vi "AddVIsToClass.vi"(8 "error in (no error)":errorcluster, 10 "Destination Folder":refnum<vi>, 11 "BaseAccessorScripter in":refnum<class "BaseAccessorScripter.lvclass">) -> (0 "error out":errorcluster, 3 "BaseAccessorScripter out":refnum<class "BaseAccessorScripter.lvclass">)   [LabVIEW 2021, in "MemberVICreation.lvlib" / "BaseAccessorScripter.lvclass"]
uses:
  <resource>/Framework/Providers/LVClassLibrary/NewAccessors/BaseAccessorScripter/BaseAccessorScripter.lvclass
  <resource>/Framework/Providers/LVClassLibrary/NewAccessors/BaseAccessorScripter/BaseAccessorScripter.lvclass/BaseAccessorScripter.ctl
  <resource>/Framework/Providers/LVClassLibrary/NewAccessors/CLSUIP_Access.ctl
  <resource>/Framework/Providers/LVClassLibrary/NewAccessors/CLSUIP_LocalizedStrings.vi
  <resource>/Framework/Providers/LVClassLibrary/NewAccessors/MemberVICreation.lvlib
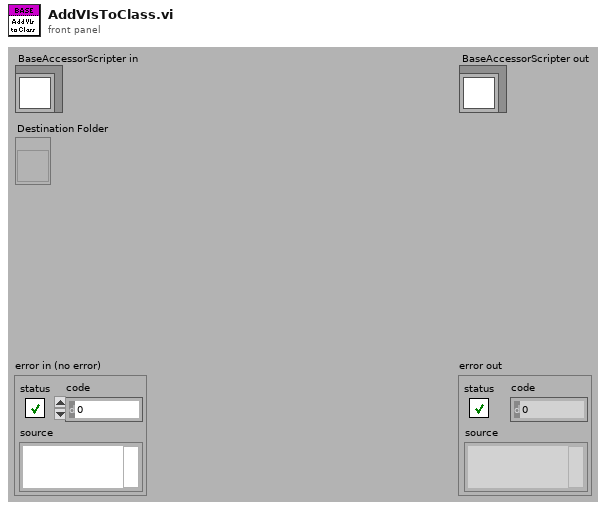
[diagram p1: front panel]
types:
  T1 = typedef "MemberVICreation.lvlib/CLSUIP_Access.ctl" = enum16{"Read", "Write", "R/W"}
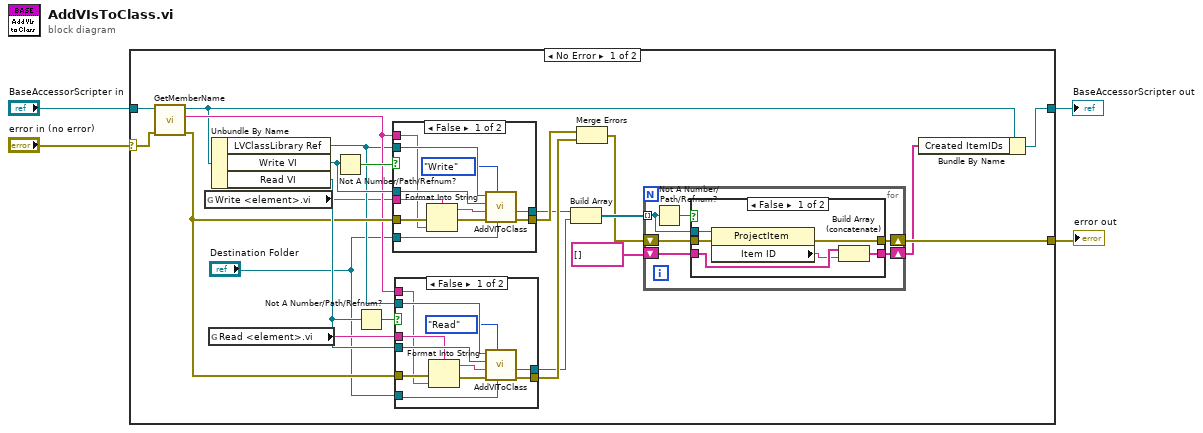
[diagram p0: block diagram]
diagram:
  n1 = case shown="No Error" "error in (no error)" {
    selector: "error in (no error)" -> [w25 w67]
    tunnel: [w7 w67] -> w3
    tunnel: [w8 w66] -> w1
    tunnel: "BaseAccessorScripter in" -> [w26 w66]
    frame No Error {
      n2 = call-dynamic "GetMemberName.vi"("error in (no error)"=w25, "BaseAccessorScripter in"=w26) -> ("error out"=w21:errorcluster, "MemberName"=w20:string, "BaseAccessorScripter out"=w9:refnum<class "BaseAccessorScripter.lvclass">)  [unwired: 7 out]
      n3 = global read "CLSUIP_LocalizedStrings.vi" "Write <element>.vi"() -> (w16:string)
      n4 = global read "CLSUIP_LocalizedStrings.vi" "Read <element>.vi"() -> (w15:string)
      n5 = Unbundle By Name(w9) -> ("LVClassLibrary Ref"=w19:refnum<vi>, "Write VI"=w24:refnum<vi>, "Read VI"=w22:refnum<vi>)
      n6 = Not A Number/Path/Refnum?(number/path/refnum=w24) -> (NaN/Path/Refnum?=w27:bool)
      n7 = Not A Number/Path/Refnum?(number/path/refnum=w22) -> (NaN/Path/Refnum?=w23:bool)
      n8 = case shown="False" w27 {
        tunnel: w20 -> [w55 _]
        tunnel: w19 -> [w64 _]
        tunnel: w24 -> [w63 _]
        tunnel: w21 -> [w60 w65]
        tunnel: [w59 w65] -> w18
        tunnel: w16 -> [w58 _]
        tunnel: [w56 _] -> w14
        tunnel: "Destination Folder" -> [w54 _]
        frame False {
          n9 = Format Into String(format string=w58, error in=w60, w55) -> (resulting string=w62:string, error out=w61:errorcluster)  [unwired: 1 in]
          n10 = call <resource>:"AddVIToClass.vi"("Destination Folder"=w54, "Access"=CLSUIP_Access."Write", "error in (no error)"=w61, "Proposed VI Name"=w62, "vi refnum in"=w63, "LVClassLibrary Ref"=w64) -> ("error out"=w59:errorcluster, "New project item ref"=w56:refnum<vi>)  [unwired: 2 in, 2 out]
        }
        frame True {
        }
      }
      n11 = case shown="False" w23 {
        tunnel: w20 -> [w42 _]
        tunnel: w19 -> [w52 _]
        tunnel: w22 -> [w51 _]
        tunnel: w21 -> [w48 w53]
        tunnel: [w47 w53] -> w17
        tunnel: w15 -> [w46 _]
        tunnel: [w44 _] -> w13
        tunnel: "Destination Folder" -> [w43 _]
        frame False {
          n12 = Format Into String(format string=w46, error in=w48, w42) -> (resulting string=w50:string, error out=w49:errorcluster)  [unwired: 1 in]
          n13 = call <resource>:"AddVIToClass.vi"("Destination Folder"=w43, "Access"=CLSUIP_Access."Read", "error in (no error)"=w49, "Proposed VI Name"=w50, "vi refnum in"=w51, "LVClassLibrary Ref"=w52) -> ("error out"=w47:errorcluster, "New project item ref"=w44:refnum<vi>)  [unwired: 2 in, 2 out]
        }
        frame True {
        }
      }
      n14 = Build Array(w14, w13) -> (w12:refnum<vi>[])
      n15 = Merge Errors(w18, w17) -> (w10:errorcluster)
      n16 = for {
        tunnel: w12 -> [w30] mode=indexing
        shift-right: [w31] -> w6
        shift-left: string[] [] -> [w32]
        shift-right: [w28] -> w7
        shift-left: w10 -> [w29]
        n17 = Not A Number/Path/Refnum?(number/path/refnum=w30) -> (NaN/Path/Refnum?=w33:bool)
        n18 = case shown="False" w33 {
          tunnel: [w38 w41] -> w31
          tunnel: w32 -> [w35 w41]
          tunnel: w30 -> [w39 _]
          tunnel: w29 -> [w37 w40]
          tunnel: [w36 w40] -> w28
          frame False {
            n19 = property class="ProjectItem"(reference=w39, error in=w37) -> (error out=w36:errorcluster, "Item ID"=w34:string)  [unwired: 1 out]
            n20 = Build Array (concatenate)(w35, w34) -> (w38:string[])
          }
          frame True {
          }
        }
      }
      n21 = Bundle By Name(cluster=w9, "Created ItemIDs"=w6) -> (w8:refnum<class "BaseAccessorScripter.lvclass">)
    }
    frame Error {
    }
  }
  "error out" <- w3
  "BaseAccessorScripter out" <- w1
